vi "NT_LL_Write Raw.vi"(8 "error in (no error)":errorcluster, 9 "unsigned byte array":u8[](array[numeric]), 10 "timestamp":u64, 11 "publishHandle":u32) -> (0 "error out":errorcluster, 3 "success":u32)   [LabVIEW 2025]
uses:
  ntcoreffi.dll
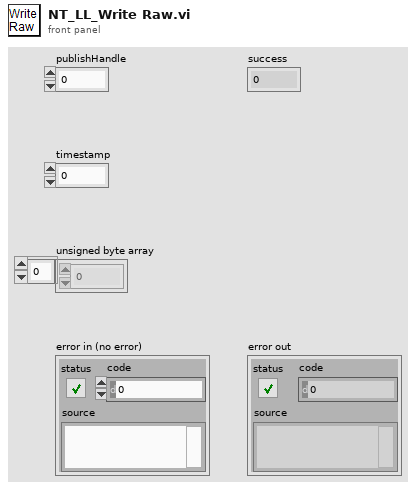
[diagram p1: front panel]
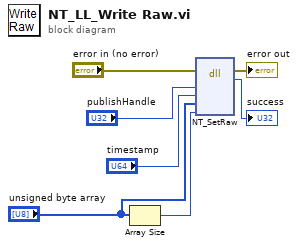
[diagram p0: block diagram]
diagram:
  n1 = Array Size(array="unsigned byte array") -> (size(s)=w5:i32)
  n2 = dll-call lib="ntcoreffi.*" fn="NT_SetRaw"(error in="error in (no error)", "publishHandle"="publishHandle", "time"="timestamp", "value"="unsigned byte array", "len"=w5) -> (error out=→"error out":errorcluster, "success"=→"success":u32)  [unwired: 6 in, 1 out]
